vi "Find Tests - When Project Contains One LVUnit Test - Returns Test Case With Path.vi"() -> ()   [LabVIEW 2017]
uses:
  LVUnit Test Discoverer/LVUnit Test Discoverer.lvclass
  LVUnit Test Discoverer.Tests.lvlib
  67af853b-47b9-474c-99b6-d22d96d58709.vi
  Test Case/Test Case.lvclass
panel:
  out "error out":errorcluster
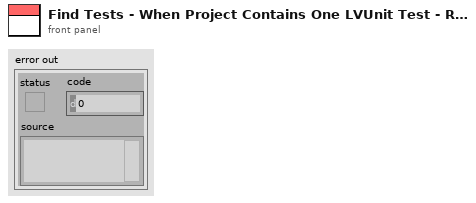
[diagram p1: front panel]
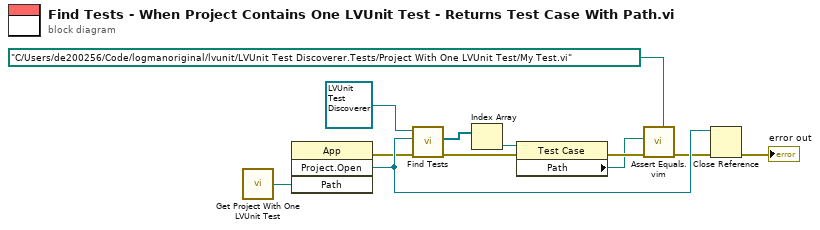
[diagram p0: block diagram]
diagram:
  n1 = call "Get Project With One LVUnit Test.vi"() -> ("Project File"=w8:path)  [unwired: 2 in]
  n2 = invoke class="App" method="Project.Open"("Path"=w8) -> (error out=w9:errorcluster, "Project:Open"=w10:refnum<vi>)  [unwired: 3 in, 2 out]
  n3 = call-dynamic "Find Tests.vi"("error in (no error)"=w9, "Project Refnum"=w10, "LVUnit Test Discoverer in"=refnum<class "LVUnit Test Discoverer.lvclass"> refnum ("LVUnit Test Discoverer")) -> ("error out"=w7:errorcluster, "Test Cases"=w5:refnum<class "Test Case.lvclass">[])  [unwired: 6 in, 1 out]
  n4 = Index Array(array=w5) -> (element=w3:refnum<class "Test Case.lvclass">)  [unwired: 1 in]
  n5 = property class="Test Case"(reference=w3, error in=w7) -> (error out=w4:errorcluster, "Path"=w2:path)  [unwired: 1 out]
  n6 = call "Assert Equals.vim"("Expected"=path "C:/Users/de200256/Code/logmanoriginal/lvunit/LVUnit Test Discoverer.Tests/Project With One LVUnit Test/My Test.vi" ("Path"), "error in (no error)"=w4, "Actual"=w2) -> ("error out"=w6:errorcluster)  [unwired: 8 in]
  n7 = Close Reference(reference=w10, error in (no error)=w6) -> (error out=→"error out":errorcluster)
